vi "construct.vi"(6 "tablecloth_type":T1 items=["Type 1", "Type 2"], 8 "error in (no error)":errorcluster, 9 "cost":dbl, 10 "id":u32) -> (0 "error out":errorcluster, 3 "ITable out":refnum<class "ITable.lvclass">)   [LabVIEW 2021]
uses:
  ITable.lvclass
  TableclothType.ctl
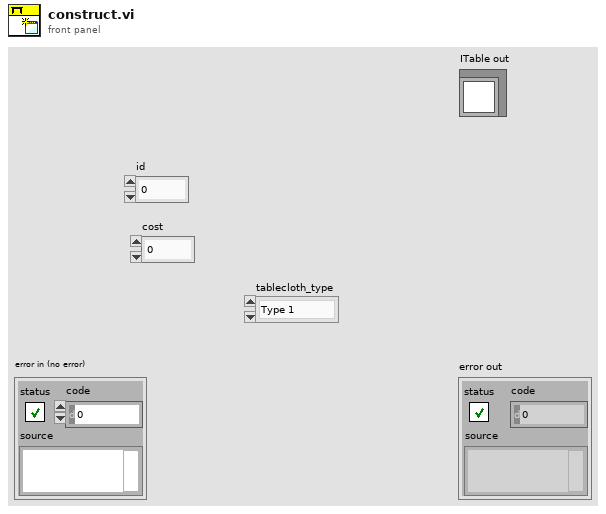
[diagram p1: front panel]
types:
  T1 = typedef "ITable.lvclass/TableclothType.ctl" = u16
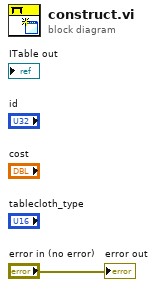
[diagram p0: block diagram]
diagram:
  "error out" <- "error in (no error)"
